vi "Move Y Raster.vi"(2 "Error In":errorcluster, 3 "Initial Direction":bool=TRUE, 4 "Y Number of Steps":string="0", 5 "Refernce In":refnum<class "_Controller.lvclass">) -> (0 "Error Out":errorcluster, 1 "Reference Out":refnum<class "_Controller.lvclass">)   [LabVIEW 2020]
doc: "Uni-axial raster scan logic for the Y direction. Moves in one direction, stopping to account for each scanning point. Once this has been completed (including any remainder steps), the motor performs the same number of total steps but in the opposite direction without stopping.\n\nArgs:\n\nReference In: Incoming communication (reference) between LabView and the scanning rig controller\nY Number of Steps: Total number of steps to move along that axis\nInitial Direction: Initial direction for the scan\nError In: Checks for any errors with the incoming communication (reference)\n\nReturns:\n\nReference Out: Output communnication (reference) between LabView and controller\nError Out: Checks for any error with output communication (reference)"
uses:
  <instrlib>/Arcus Ethernet Driver 1.0.0/ArcusEthernetComm/classes/Controller/_Controller.lvclass
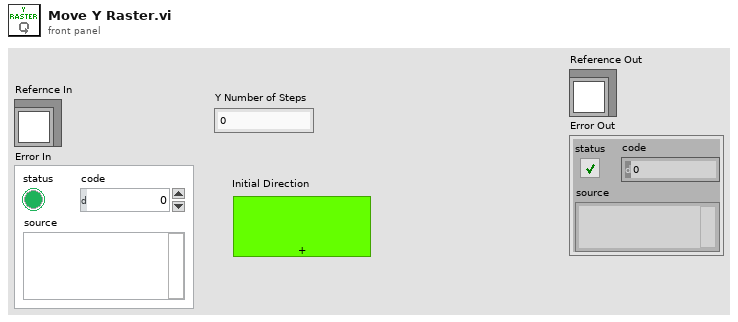
[diagram p1: front panel]
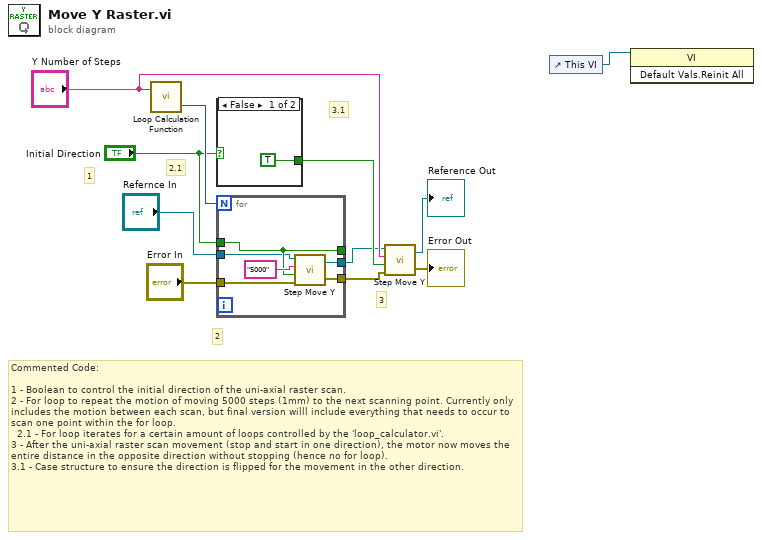
[diagram p0: block diagram]
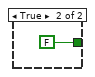
[diagram p2: hidden frame]
diagram:
  # "3.1"
  # "3"
  # "2.1"
  # "2"
  # "1"
  # "Commented Code:\n\n1 - Boolean to control the initial direction of the uni-axial raster scan.\n2 - For loop to repeat the motion of moving 5000 steps (1mm) to the next scanning point. Currently only includes the motion between each scan, but final version willl include everything that needs to occur to scan one point within the for loop.\n  2.1 - For loop iterates for a certain amount of loops controlled by the 'loop_calculator.vi'.\n3 - After the uni-axial raster scan movement (stop and start in one direction), the motor now moves the entire distance in the opposite direction without stopping (hence no for loop).\n3.1 - Case structure to ensure the direction is flipped for the movement in the other direction."
  n1 = call "Loop Calculation Function.vi"("Number of Steps"="Y Number of Steps") -> ("No. of Scan Points"=w11:i32)  [unwired: 1 in, 1 out]
  n2 = case shown="False" "Initial Direction" {
    tunnel: [TRUE FALSE] -> w4
    frame False {
    }
    frame True {
    }
  }
  n3 = for {
    N: w11 -> [_]
    tunnel: [w19] -> w2
    tunnel: "Initial Direction" -> [w16]
    tunnel: [w18] -> w1
    tunnel: [w16] -> _
    tunnel: "Refernce In" -> [w15]
    tunnel: "Error In" -> [w14]
    n4 = call "Step Move Y.vi"("Error In"=w14, "Direction"=w16, "No. of Y Steps"="5000" ("X Steps"), "Reference In"=w15) -> ("Error Out"=w18:errorcluster, "Reference Out"=w19:refnum<class "_Controller.lvclass">)
  }
  n5 = call "Step Move Y.vi"("Error In"=w1, "Direction"=w4, "No. of Y Steps"="Y Number of Steps", "Reference In"=w2) -> ("Error Out"=→"Error Out":errorcluster, "Reference Out"=→"Reference Out":refnum<class "_Controller.lvclass">)
  n6 = control-ref of="This VI"() -> (w3:refnum<vi>)
  n7 = invoke class="VI" method="Default Vals.Reinit All"(reference=w3) -> ()  [unwired: 2 in, 3 out]
